vi "DSF.Transceiver.UDP.Settings.Transfer Group.vi"(8 "error in (no error)":errorcluster, 10 "Transfer Groups Configurations":refnum<class "DSF.Shared.Configuration.Transfer Group.lvclass">[](array[class]), 11 "UDP Transceiver in":refnum<class "DSF.Transceiver.UDP.lvclass">) -> (0 "error out":errorcluster, 2 "Transfer Group parameters":T1[](array[typedef]) {"Rx"."max size" format="%d bytes"; "Rx"."Transfers Rx"."source address" format="%d ms"; "Rx"."Transfers Rx"."timeout" format="%d bytes"}, 3 "UDP Transceiver out":refnum<class "DSF.Transceiver.UDP.lvclass">)   [LabVIEW 2017, in "DSF.Transceiver.UDP.lvlib" / "DSF.Transceiver.UDP.lvclass"]
uses:
  DSF.Transceiver.UDP.lvclass
  DSF.Transceiver.UDP.Parameters.Transfer Group.ctl
  DSF.Transceiver.UDP.Parameters.Transfer Group.Rx.ctl
  DSF.Transceiver.UDP.Parameters.Transfer.Rx.ctl
  DSF.Transceiver.UDP.Parameters.Transfer Group.Tx.ctl
  DSF.Transceiver.UDP.Parameters.Transfer.Tx.ctl
  DSF Core/Built/Engine/DSF.Engine.lvlibp/Shared/Classes/Transfer Group/DSF.Shared.Configuration.Transfer Group.lvclass
  DSF.Transceiver.UDP.lvclass/DSF.Transceiver.UDP.ctl
  DSF Core/Built/Engine/DSF.Engine.lvlibp/Shared/Classes/Configuration/DSF.Shared.Configuration.lvclass
  DSF Core/Built/Engine/DSF.Engine.lvlibp/Shared/Classes/Transfer/DSF.Shared.Configuration.Transfer.lvclass
  C:/Git/DSF/DSF Core/Built/Engine/DSF.Engine.lvlibp/Shared/Classes/Configuration/DSF.Shared.Configuration.lvclass
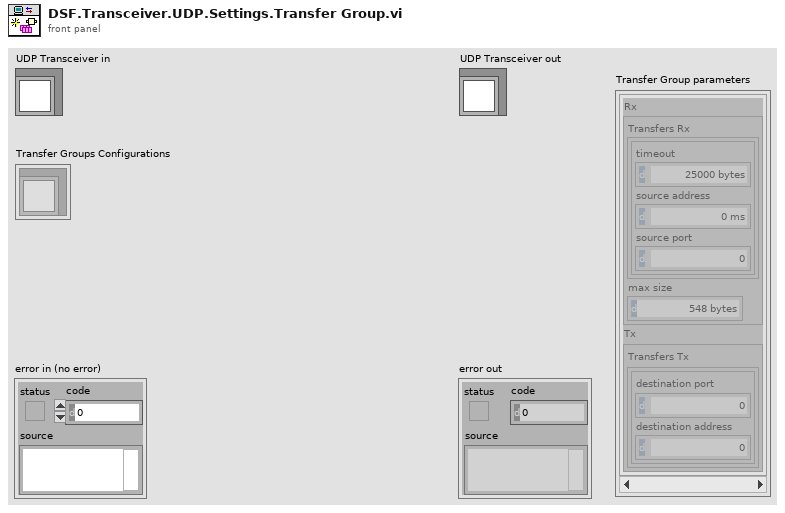
[diagram p1: front panel]
types:
  T1 = typedef "DSF.Transceiver.UDP.lvlib/DSF.Transceiver.UDP.lvclass/DSF.Transceiver.UDP.Parameters.Transfer Group.ctl" = cluster{"Rx":T2, "Tx":T4}
  T2 = typedef "DSF.Transceiver.UDP.lvlib/DSF.Transceiver.UDP.lvclass/DSF.Transceiver.UDP.Parameters.Transfer Group.Rx.ctl" = cluster{"Transfers Rx":T3[], "max size":i32}
  T3 = typedef "DSF.Transceiver.UDP.lvlib/DSF.Transceiver.UDP.lvclass/DSF.Transceiver.UDP.Parameters.Transfer.Rx.ctl" = cluster{"timeout":i32, "source address":u32, "source port":u16}
  T4 = typedef "DSF.Transceiver.UDP.lvlib/DSF.Transceiver.UDP.lvclass/DSF.Transceiver.UDP.Parameters.Transfer Group.Tx.ctl" = cluster{"Transfers Tx":T5[]}
  T5 = typedef "DSF.Transceiver.UDP.lvlib/DSF.Transceiver.UDP.lvclass/DSF.Transceiver.UDP.Parameters.Transfer.Tx.ctl" = cluster{"destination port":u16, "destination address":u32}
  T6 = typedef "DSF.Engine.lvlibp/DSF Configuration API.lvlib/DSF Direction.ctl" = enum8{"Tx", "Rx"}
  T7 = typedef "DSF.Engine.lvlibp/DSF Configuration API.lvlib/DSF Settings Info.ctl" = cluster{"key":string, "value":string}[]
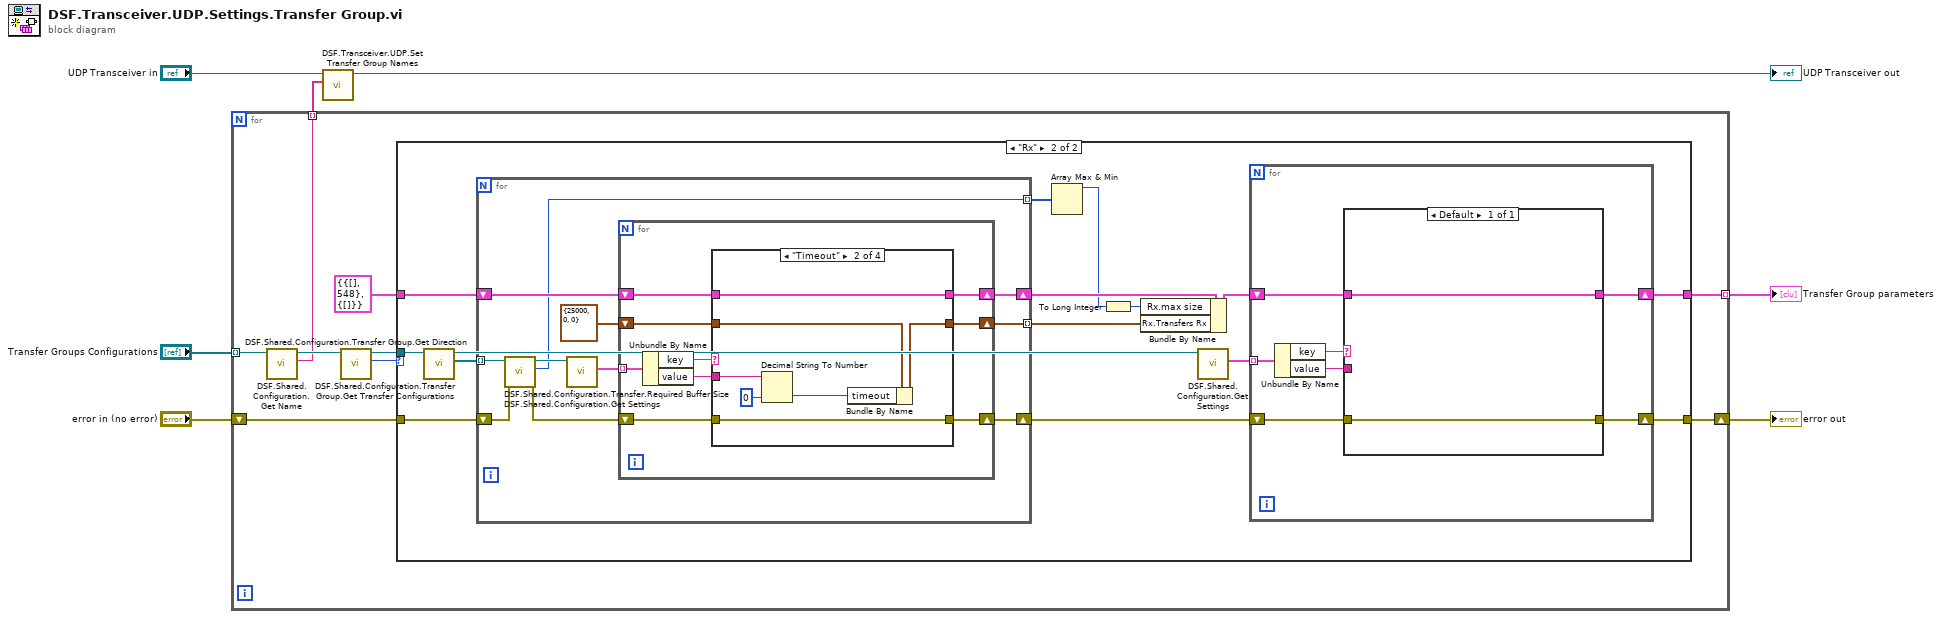
[diagram p0: block diagram]
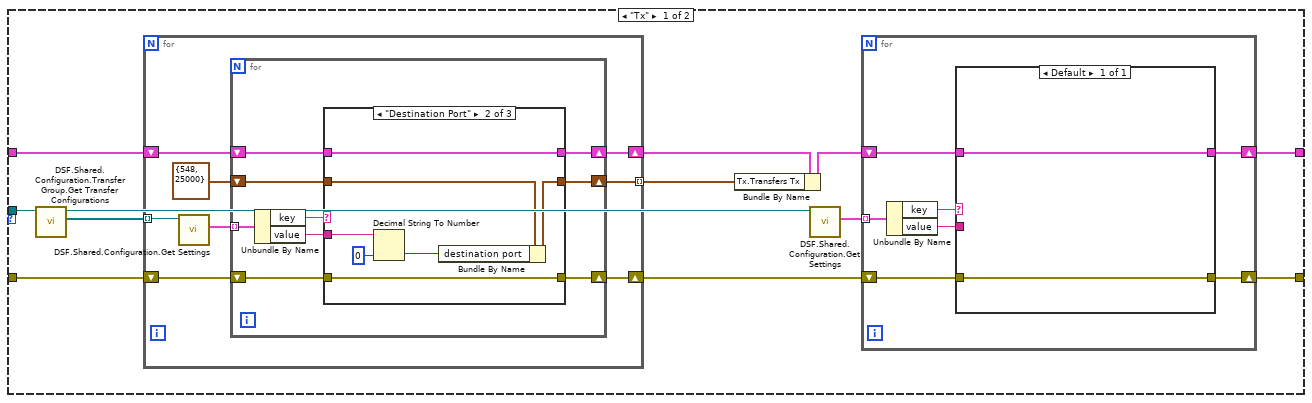
[diagram p2: hidden frame]
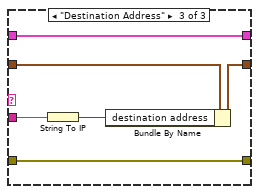
[diagram p4: hidden frame]
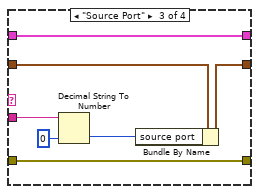
[diagram p6: hidden frame]
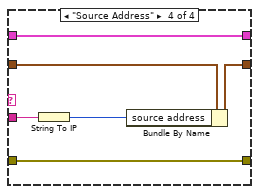
[diagram p7: hidden frame]
diagram:
  n1 = for {
    tunnel: "Transfer Groups Configurations" -> [w8] mode=indexing
    tunnel: [w15] -> w3 mode=indexing
    tunnel: [w12] -> w4 mode=indexing
    shift-right: [w10] -> w5
    shift-left: "error in (no error)" -> [w11]
    n2 = call "DSF.Shared.Configuration.Get Name.vi"("Configuration in"=w8) -> ("name"=w15:string, "Configuration out"=w16:refnum<class "DSF.Shared.Configuration.Transfer Group.lvclass">)  [unwired: 9 in]
    n3 = call "DSF.Shared.Configuration.Transfer Group.Get Direction.vi"("Transfer Group Configuration in"=w16) -> ("direction"=w13:T6, "Transfer Group Configuration out"=w14:refnum<class "DSF.Shared.Configuration.Transfer Group.lvclass">)  [unwired: 9 in]
    n4 = case shown="\"Rx\"" w13 {
      tunnel: w14 -> [w22 w77]
      tunnel: T1 {"Rx"={"Transfers Rx"=[], "max size"=548}, "Tx"={"Transfers Tx"=[]}} ("Rx/Tx Parameters") -> [w23 w78]
      tunnel: [w27 w85] -> w12
      tunnel: w11 -> [w25 w79]
      tunnel: [w26 w84] -> w10
      frame "Tx" {
        n5 = call "DSF.Shared.Configuration.Transfer Group.Get Transfer Configurations.vi"("Transfer Group Configuration in"=w22) -> ("Transfer Configurations"=w20:refnum<class "DSF.Shared.Configuration.Transfer.lvclass">[], "Transfer Group Configuration out"=w21:refnum<class "DSF.Shared.Configuration.Transfer Group.lvclass">)  [unwired: 9 in]
        n6 = for {
          shift-right: [w35] -> w19
          shift-left: w23 -> [w36]
          shift-right: [w33] -> w24
          shift-left: w25 -> [w34]
          tunnel: w20 -> [w32] mode=indexing
          tunnel: [w29] -> w18 mode=indexing
          n7 = call "DSF.Shared.Configuration.Get Settings.vi"("Configuration in"=w32) -> ("settings"=w31:T7)  [unwired: 9 in, 1 out]
          n8 = for {
            tunnel: w31 -> [w39] mode=indexing
            shift-right: [w42] -> w35
            shift-left: w36 -> [w43]
            shift-right: [w40] -> w33
            shift-left: w34 -> [w41]
            shift-right: [w38] -> w29
            shift-left: T5 {"destination port"=548, "destination address"=25000} ("Transfer Tx") -> [w37]
            n9 = Unbundle By Name(w39) -> ("key"=w45:string, "value"=w44:string)
            n10 = case shown="\"Destination Port\"" w45 {
              tunnel: w44 -> [_ w55 w60]
              tunnel: w43 -> [w48 w50 w57]
              tunnel: [w48 w50 w57] -> w42
              tunnel: w41 -> [w47 w52 w61]
              tunnel: [w47 w52 w61] -> w40
              tunnel: w37 -> [w46 w51 w58]
              tunnel: [w46 w49 w56] -> w38
              frame Default {
              }
              frame "Destination Port" {
                n11 = Decimal String To Number(string=w55, default (0L)=u16 0 ("default (0 I32)")) -> (number=w53:u16)  [unwired: 1 in, 1 out]
                n12 = Bundle By Name(cluster=w51, "destination port"=w53) -> (w49:T5)
              }
              frame "Destination Address" {
                n13 = String To IP(1:w60) -> (0:w59:u32)
                n14 = Bundle By Name(cluster=w58, "destination address"=w59) -> (w56:T5)
              }
            }
          }
        }
        n15 = Bundle By Name(cluster=w19, "Tx.Transfers Tx"=w18) -> (w17:T1)
        n16 = call "DSF.Shared.Configuration.Get Settings.vi"("Configuration in"=w21) -> ("settings"=w28:T7)  [unwired: 9 in, 1 out]
        n17 = for {
          tunnel: w28 -> [w66] mode=indexing
          shift-right: [w64] -> w27
          shift-left: w17 -> [w65]
          shift-right: [w62] -> w26
          shift-left: w24 -> [w63]
          n18 = Unbundle By Name(w66) -> ("key"=w68:string, "value"=w67:string)
          n19 = case shown="Default" w68 {
            tunnel: w67 -> [_]
            tunnel: w65 -> [w70]
            tunnel: [w70] -> w64
            tunnel: w63 -> [w69]
            tunnel: [w69] -> w62
            frame Default {
            }
          }
        }
      }
      frame "Rx" {
        n20 = call "DSF.Shared.Configuration.Transfer Group.Get Transfer Configurations.vi"("Transfer Group Configuration in"=w77) -> ("Transfer Configurations"=w82:refnum<class "DSF.Shared.Configuration.Transfer.lvclass">[], "Transfer Group Configuration out"=w83:refnum<class "DSF.Shared.Configuration.Transfer Group.lvclass">)  [unwired: 9 in]
        n21 = for {
          shift-right: [w95] -> w81
          shift-left: w78 -> [w96]
          shift-right: [w94] -> w74
          shift-left: w79 -> [w88]
          tunnel: w82 -> [w90] mode=indexing
          tunnel: [w91] -> w80 mode=indexing
          tunnel: [w86] -> w73 mode=indexing
          n22 = call "DSF.Shared.Configuration.Transfer.Required Buffer Size.vi"("error in (no error)"=w88, "Transfer Configuration in"=w90) -> ("error out"=w87:errorcluster, "required buffer size"=w86:u64, "Transfer Configuration out"=w89:refnum<class "DSF.Shared.Configuration.Transfer.lvclass">)  [unwired: 7 in]
          n23 = call "DSF.Shared.Configuration.Get Settings.vi"("Configuration in"=w89) -> ("settings"=w93:T7)  [unwired: 9 in, 1 out]
          n24 = for {
            tunnel: w93 -> [w99] mode=indexing
            shift-right: [w102] -> w95
            shift-left: w96 -> [w103]
            shift-right: [w100] -> w94
            shift-left: w87 -> [w101]
            shift-right: [w98] -> w91
            shift-left: T3 {"timeout"=25000, "source address"=0, "source port"=0} ("Transfer Rx") -> [w97]
            n25 = Unbundle By Name(w99) -> ("key"=w105:string, "value"=w104:string)
            n26 = case shown="\"Timeout\"" w105 {
              tunnel: w104 -> [_ w115 w122 w124]
              tunnel: w103 -> [w108 w110 w117 w126]
              tunnel: [w108 w110 w117 w126] -> w102
              tunnel: w101 -> [w107 w112 w119 w128]
              tunnel: [w107 w112 w119 w128] -> w100
              tunnel: w97 -> [w106 w111 w118 w127]
              tunnel: [w106 w109 w116 w125] -> w98
              frame Default {
              }
              frame "Timeout" {
                n27 = Decimal String To Number(string=w115, default (0L)=0 ("default (0 I32)")) -> (number=w113:i32)  [unwired: 1 in, 1 out]
                n28 = Bundle By Name(cluster=w111, "timeout"=w113) -> (w109:T3)
              }
              frame "Source Port" {
                n29 = Decimal String To Number(string=w122, default (0L)=u16 0 ("default (0 I32)")) -> (number=w120:u16)  [unwired: 1 in, 1 out]
                n30 = Bundle By Name(cluster=w118, "source port"=w120) -> (w116:T3)
              }
              frame "Source Address" {
                n31 = String To IP(1:w124) -> (0:w123:u32)
                n32 = Bundle By Name(cluster=w127, "source address"=w123) -> (w125:T3)
              }
            }
          }
        }
        n33 = Array Max & Min(array=w73) -> (max value=w72:u64)  [unwired: 3 out]
        n34 = To Long Integer(number=w72) -> (32bit integer=w71:i32)
        n35 = Bundle By Name(cluster=w81, "Rx.max size"=w71, "Rx.Transfers Rx"=w80) -> (w76:T1)
        n36 = call "DSF.Shared.Configuration.Get Settings.vi"("Configuration in"=w83) -> ("settings"=w75:T7)  [unwired: 9 in, 1 out]
        n37 = for {
          tunnel: w75 -> [w133] mode=indexing
          shift-right: [w131] -> w85
          shift-left: w76 -> [w132]
          shift-right: [w129] -> w84
          shift-left: w74 -> [w130]
          n38 = Unbundle By Name(w133) -> ("key"=w135:string, "value"=w134:string)
          n39 = case shown="Default" w135 {
            tunnel: w134 -> [_]
            tunnel: w132 -> [w137]
            tunnel: [w137] -> w131
            tunnel: w130 -> [w136]
            tunnel: [w136] -> w129
            frame Default {
            }
          }
        }
      }
    }
  }
  "error out" <- w5
  "Transfer Group parameters" <- w4
  n40 = call "DSF.Transceiver.UDP.Set Transfer Group Names.vi"("Transfer Group names"=w3, "UDP Transceiver in"="UDP Transceiver in") -> ("UDP Transceiver out"=→"UDP Transceiver out":refnum<class "DSF.Transceiver.UDP.lvclass">)  [unwired: 9 in]
